vi "Get FilePath.vi"(8 "error in (no error)":errorcluster, 11 "Document in":refnum<class "Document.lvclass">) -> (0 "error out":errorcluster, 2 "FilePath":path, 3 "Document out":refnum<class "Document.lvclass">)   [LabVIEW 2020, in "LabVIEW NPOI.lvlib" / "Document.lvclass"]
doc: "Gets the <b>File Path</b> from the <b>Document</b>."
uses:
  Document.lvclass
  Document.lvclass/Document.ctl
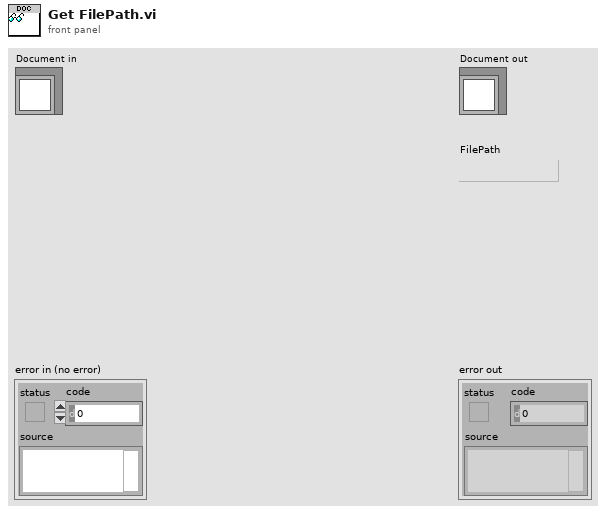
[diagram p1: front panel]
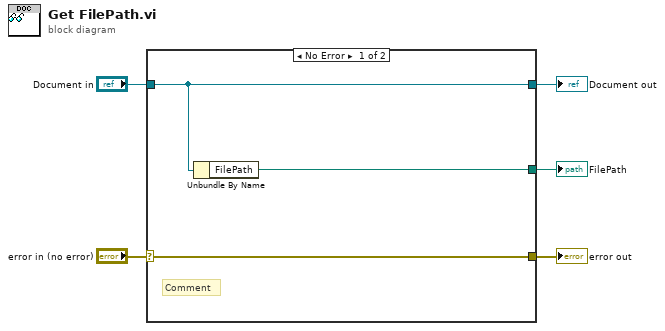
[diagram p0: block diagram]
diagram:
  n1 = case shown="No Error" "error in (no error)" {
    selector: "error in (no error)" -> [w8 w9]
    tunnel: [w8 w9] -> w4
    tunnel: [w7 w10] -> w2
    tunnel: "Document in" -> [w7 w10]
    tunnel: [w6 _] -> w1
    frame No Error {
      # "Comment"
      n2 = Unbundle By Name(w7) -> ("FilePath"=w6:path)
    }
    frame Error {
    }
  }
  "error out" <- w4
  "Document out" <- w2
  "FilePath" <- w1
